vi "Setup.vi"(8 "error in (no error)":errorcluster, 11 "Scan Driver in":refnum<class "Scan Driver.lvclass">) -> (0 "error out":errorcluster, 3 "Scan Driver out":refnum<class "Scan Driver.lvclass">)   [LabVIEW 2017, in "Scan Driver.lvclass"]
doc: "GUI constructor for new Scan Driver instances. Call the component objects' Setup UI methods and use their GUIs to construct them too."
uses:
  Scan Driver.lvclass
  Scan Driver.lvclass/Scan Driver.ctl
  Scanners/Double Scanner/Double Scanner.lvclass
  C:/LabVIEW-programs/Scanners/Scanner/Scanner.lvclass
  Data Processing/Multi/Multi.lvclass
  C:/LabVIEW-programs/Data Processing/Aux Data Source/Aux Data Source.lvclass
  Readers/Reader/Reader.lvclass
  Scanners/Scanner/Scanner.lvclass
  File IO/File IO.lvclass
panel:
  in  "?":bool
  in  "Constant":dbl=1.0
  in  "Time between scans":dbl[unit]
  in  "Cancel":bool
  in  "# Scans":u32=1
  in  "Start Scan":bool
  in  "Aux Data Sources":T1
  # "Generic Scan Setup"
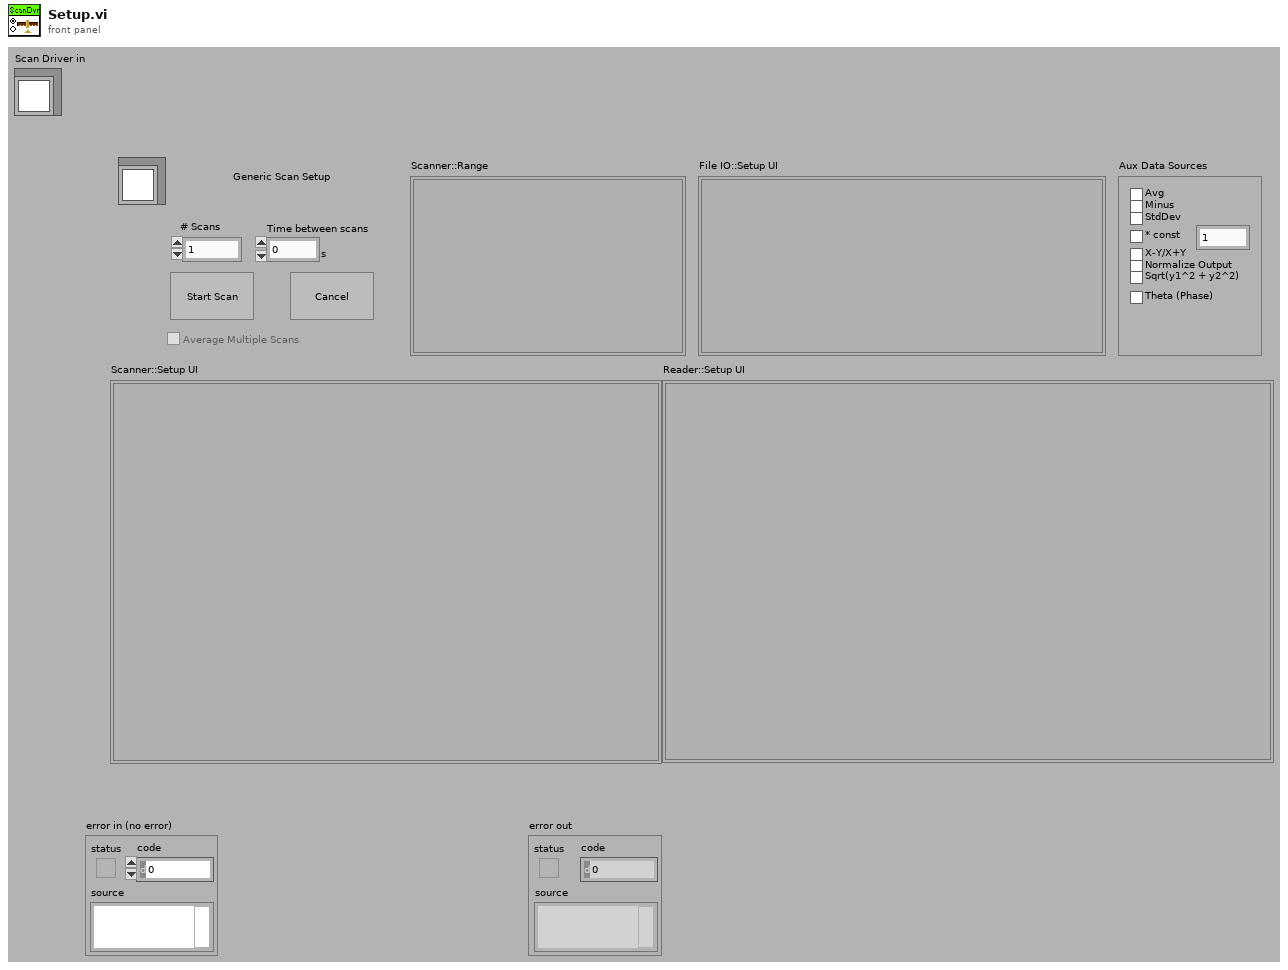
[diagram p1: front panel]
types:
  T1 = cluster{"Avg":bool, "Minus":bool, "StdDev":bool, "* const":bool, "X-Y/X+Y":bool, "Normalize Output":bool, "Sqrt(y1^2 + y2^2)":bool, "Theta (Phase)":bool}
  T2 = typedef "Scan Driver.lvclass/Scan Setup Mode.ctl" = enum32{"New Scan", "Load Last Scan", "Load Scan:"}
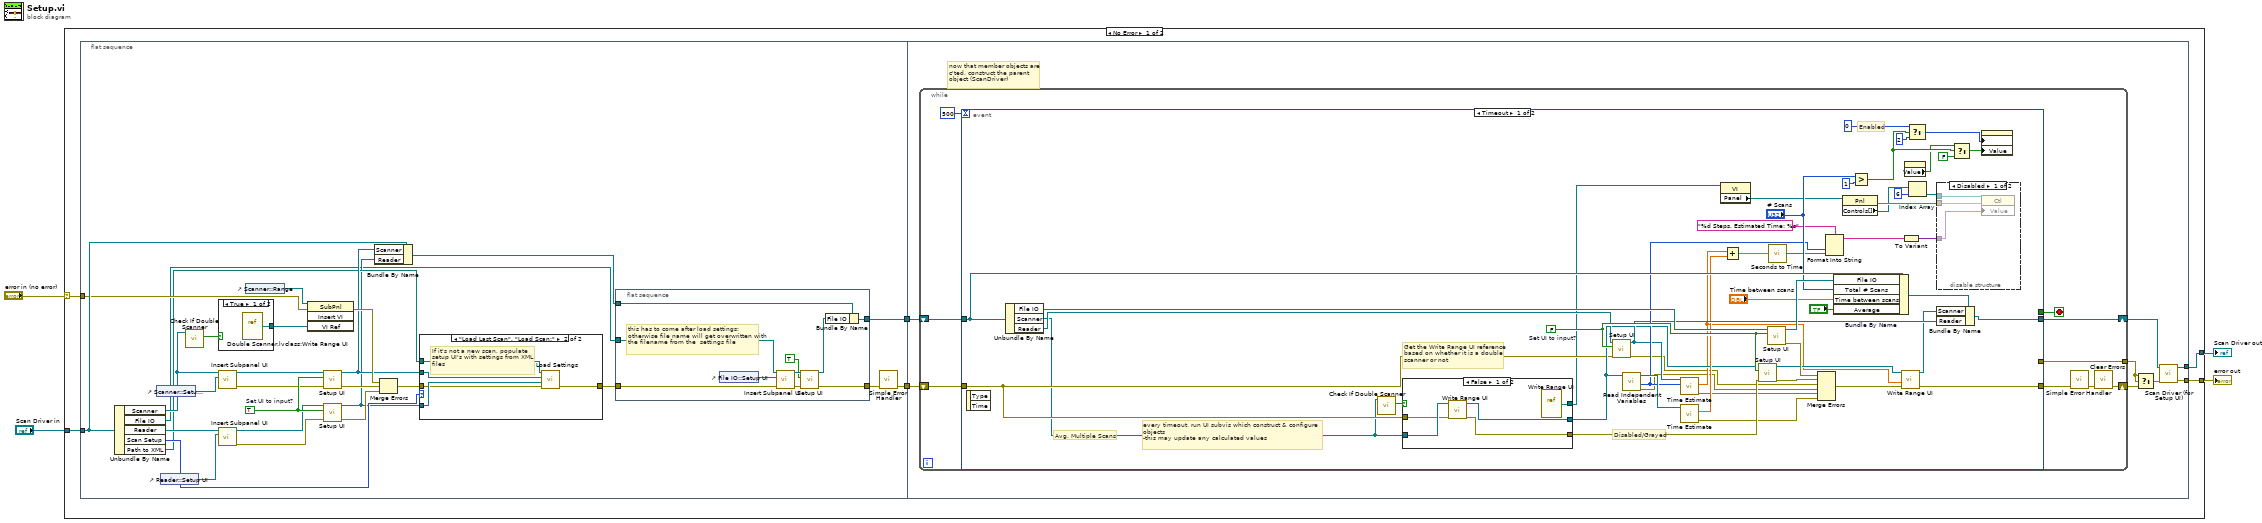
[diagram p0: block diagram]
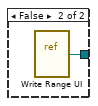
[diagram p3: hidden frame]
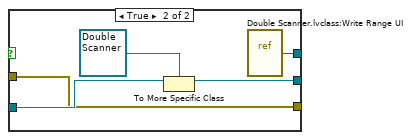
[diagram p5: hidden frame]
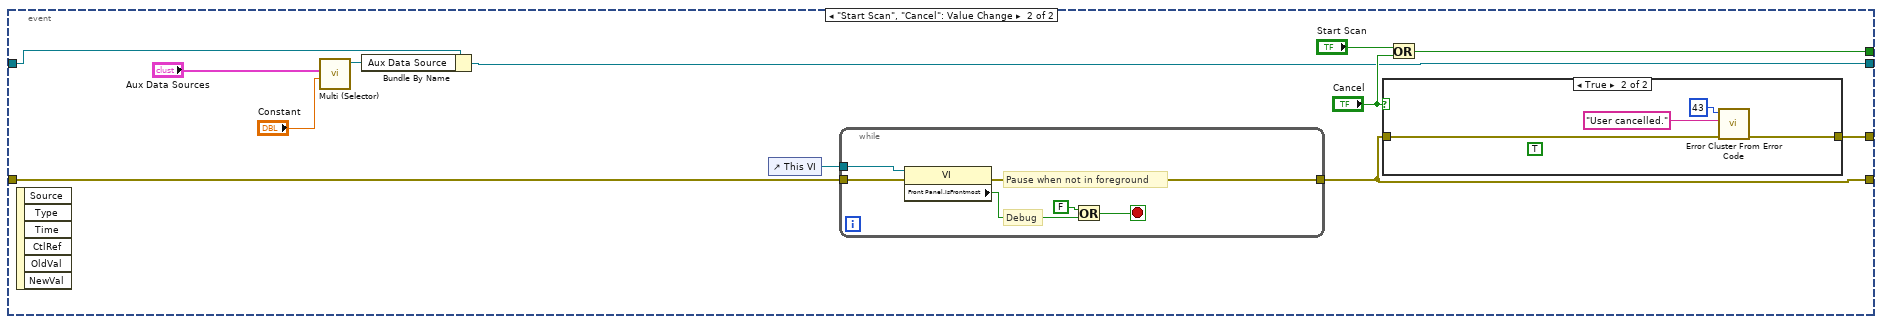
[diagram p6: hidden frame]
diagram:
  n1 = case shown="No Error" "error in (no error)" {
    selector: "error in (no error)" -> [w10 w160]
    tunnel: [w9 w160] -> w3
    tunnel: [w5 w159] -> w1
    tunnel: "Scan Driver in" -> [w8 w159]
    frame No Error {
      n2 = flat-sequence {
        tunnel: w10 -> [w27]
        tunnel: w8 -> [w30]
        tunnel: [w36] -> w7
        tunnel: [w14] -> w6
        tunnel: [w59] -> w9
        tunnel: w7 -> [w64]
        tunnel: w6 -> [w63]
        tunnel: [w57] -> w5
        frame #0 {
          w35 = TRUE  # Set UI to input?
          n3 = Unbundle By Name(w30) -> ("Scanner"=w22:refnum<class "Scanner.lvclass">, "File IO"=w13:refnum<class "File IO.lvclass">, "Reader"=w21:refnum<class "Reader.lvclass">, "Scan Setup"=w20:T2, "Path to XML"=w18:path)
          n4 = control-ref of="Scanner::Setup UI"() -> (w38:refnum<vi>)
          n5 = control-ref of="Reader::Setup UI"() -> (w37:refnum<vi>)
          n6 = call "Check If Double Scanner.vi"("Scanner in"=w22) -> ("Is Double Scanner?"=w29:bool)  [unwired: 10 in]
          n7 = case shown="True" w29 {
            tunnel: [w55 w56] -> w26
            frame True {
              n8 = vi-ref "Double Scanner.lvclass:Write Range UI.vi"() -> (w55:refnum<vi>)
            }
            frame False {
              n9 = vi-ref "Write Range UI.vi"() -> (w56:refnum<vi>)
            }
          }
          n10 = call "Insert Subpanel UI.vi"("Subpanel in"=w38, "LabVIEW Object"=w22) -> ("error out"=w32:errorcluster, "LabVIEW Object out"=w31:refnum<class "Scanner.lvclass">)  [unwired: 1 in, 7 out]
          n11 = call "Insert Subpanel UI.vi"("Subpanel in"=w37, "LabVIEW Object"=w21) -> ("error out"=w33:errorcluster, "LabVIEW Object out"=w34:refnum<class "Reader.lvclass">)  [unwired: 1 in, 7 out]
          n12 = control-ref of="Scanner::Range"() -> (w28:refnum<vi>)
          n13 = invoke on="Invoke Node" class="SubPnl" method="Insert VI"(reference=w28, error in=w27, "VI Ref"=w26) -> (error out=w25:errorcluster)  [unwired: 1 in, 3 out]
          n14 = call-dynamic "Setup UI.vi"("error in (no error)"=w32, "Set UI to input? (F)"=w35, "Scanner in"=w31) -> ("error out"=w24:errorcluster, "Scanner out"=w19:refnum<class "Scanner.lvclass">)  [unwired: 7 out]
          n15 = call-dynamic "Setup UI.vi"("error in (no error)"=w33, "Set UI to input? (F)"=w35, "Reader in"=w34) -> ("error out"=w23:errorcluster, "Reader out"=w17:refnum<class "Reader.lvclass">)  [unwired: 1 in, 6 out]
          n16 = Bundle By Name(cluster=w30, "Scanner"=w19, "Reader"=w17) -> (w15:refnum<class "Scan Driver.lvclass">)
          n17 = Merge Errors(w25, w24, w23) -> (w16:errorcluster)
          n18 = case shown="\"Load Last Scan\", \"Load Scan:\"" w20 {
            tunnel: w19 -> [_ w54]
            tunnel: w18 -> [_ w53]
            tunnel: w17 -> [_ w52]
            tunnel: w16 -> [w49 w51]
            tunnel: [w49 w50] -> w12
            frame "New Scan", Default {
            }
            frame "Load Last Scan", "Load Scan:" {
              # "If it's not a new scan, populate setup UI's with settings from XML files"
              n19 = call "Load Settings.vi"("error in (no error)"=w51, "Reader Object"=w52, "Scanner Object"=w54, "XML File Path"=w53) -> ("error out"=w50:errorcluster)  [unwired: 7 in]
            }
          }
          n20 = flat-sequence {
            tunnel: w15 -> [w46]
            tunnel: [w45] -> w14
            tunnel: w13 -> [w44]
            tunnel: w12 -> [w40]
            tunnel: [w39] -> w11
            frame #0 {
              # "this has to come after load settings; otherwise file name will get overwritten with the filename from the  settings file"
              n21 = control-ref of="File IO::Setup UI"() -> (w48:refnum<vi>)
              n22 = call "Insert Subpanel UI.vi"("error in (no error)"=w40, "Subpanel in"=w48, "LabVIEW Object"=w44) -> ("error out"=w43:errorcluster, "LabVIEW Object out"=w47:refnum<class "File IO.lvclass">)  [unwired: 7 out]
              n23 = call-dynamic "Setup UI.vi"("error in (no error)"=w43, "Set UI to input?"=TRUE, "File IO in"=w47) -> ("error out"=w39:errorcluster, "File IO out"=w42:refnum<class "File IO.lvclass">)  [unwired: 7 out]
              n24 = Bundle By Name(cluster=w46, "File IO"=w42) -> (w45:refnum<class "Scan Driver.lvclass">)
            }
          }
          n25 = call <vilib>:"Simple Error Handler.vi"("error in (no error)"=w11) -> ("error out"=w36:errorcluster)  [unwired: 1 in, 7 out]
        }
        frame #1 {
          # "now that member objects are\nc'ted, construct the parent\nobject (ScanDriver)"
          n26 = while {
            shift-right: [w72] -> w61
            shift-left: w64 -> [w73]
            shift-right: [w65] -> w58
            shift-left: w63 -> [w71]
            tunnel: [w67] -> w62
            stop <- w66 stop-if-true
            n27 = event shown="[0] Timeout" {
              selector: _ -> [_ _]
              dyn-events: _ -> [_ _]
              timeout: 500 -> [_ _]
              tunnel: w73 -> [w87 w138]
              tunnel: [w80 w136] -> w70
              tunnel: w71 -> [w121 w143]
              tunnel: [w122 w142] -> w65
              tunnel: [_ w144] -> w66
              tunnel: [_ w147] -> w67
              event Timeout {
                w119 = FALSE  # Set UI to input?
                # "Get the Write Range UI reference\nbased on whether it is a double\nscanner or not"
                # "Avg. Multiple Scans"
                # "Disabled/Grayed"
                # "Enabled"
                # "every timeout, run UI subvis which construct & configure objects\n-this may update any calculated values"
                n28 = event-data() -> ()  [unwired: 3 out]
                n29 = Unbundle By Name(w121) -> ("File IO"=w118:refnum<class "File IO.lvclass">, "Scanner"=w85:refnum<class "Scanner.lvclass">, "Reader"=w113:refnum<class "Reader.lvclass">)
                n30 = call "Check If Double Scanner.vi"("Scanner in"=w85) -> ("Is Double Scanner?"=w86:bool)  [unwired: 10 in]
                n31 = case shown="False" w86 {
                  tunnel: w85 -> [w130 w135]
                  tunnel: [w129 w132] -> w89
                  tunnel: [w128 w131] -> w88
                  tunnel: w87 -> [w127 w131]
                  tunnel: [w126 w133] -> w84
                  frame False {
                    n32 = call-dynamic "Write Range UI.vi"("error in (no error)"=w127, "Scanner in"=w130) -> ("error out"=w128:errorcluster, "Scanner out"=w129:refnum<class "Scanner.lvclass">)  [unwired: 2 in, 6 out]
                    n33 = vi-ref "Write Range UI.vi"() -> (w126:refnum<vi>)
                  }
                  frame True {
                    n34 = To More Specific Class(target class=refnum<class "Double Scanner.lvclass"> refnum ("Double Scanner.lvclass"), reference=w135) -> (specific class reference=w132:refnum<class "Double Scanner.lvclass">)  [unwired: 1 in, 1 out]
                    n35 = vi-ref "Double Scanner.lvclass:Write Range UI.vi"() -> (w133:refnum<vi>)
                  }
                }
                n36 = call-dynamic "Setup UI.vi"("error in (no error)"=w87, "Set UI to input? (F)"=w119, "Reader in"=w113) -> ("error out"=w77:errorcluster, "Reader out"=w93:refnum<class "Reader.lvclass">)  [unwired: 1 in, 6 out]
                n37 = call-dynamic "Read Independent Variables.vi"("Scanner.lvclass in"=w89) -> ("error out"=w76:errorcluster, "size"=w94:i32, "Scanner.lvclass out"=w95:refnum<class "Scanner.lvclass">)  [unwired: 1 in, 7 out]
                n38 = call-dynamic "Time Estimate.vi"("Points"=w94, "Reader in"=w93) -> ("error out"=w75:errorcluster, "time"=w78:dbl[unit])  [unwired: 7 in, 1 out]
                n39 = call-dynamic "Time Estimate.vi"("Scanner.lvclass"=w95) -> ("error out"=w74:errorcluster, "time"=w92:dbl[unit])  [unwired: 7 in, 2 out]
                n40 = property class="VI"(reference=w84) -> ("Panel"=w99:refnum<vi>)  [unwired: 1 in, 2 out]
                n41 = Add(x=w78, y=w92) -> (x+y=w91:dbl[unit])
                n42 = call-dynamic "Setup UI.vi"("error in (no error)"=w88, "Set UI to input? (F)"=w119, "Scanner in"=w89) -> ("error out"=w114:errorcluster, "Scanner out"=w83:refnum<class "Scanner.lvclass">)  [unwired: 7 out]
                n43 = call-dynamic "Setup UI.vi"("Set UI to input?"=w119, "File IO in"=w118) -> ("error out"=w116:errorcluster, "File IO out"=w117:refnum<class "File IO.lvclass">)  [unwired: 1 in, 7 out]
                n44 = call "Seconds to Time.vi"("Seconds"=w91) -> ("Time"=w96:string)
                n45 = Merge Errors(w116, w114, w77, w76, w75, w74) -> (w81:errorcluster)
                n46 = Format Into String(format string="%d Steps, Estimated Time: %s", w94, w96) -> (resulting string=w90:string)  [unwired: 2 in, 1 out]
                n47 = Bundle By Name(cluster=w121, "File IO"=w117, "Total # Scans"="# Scans", "Time between scans"="Time between scans", "Average"="?") -> (w120:refnum<class "Scan Driver.lvclass">)
                n48 = property class="Pnl"(reference=w99) -> (error out=w100:errorcluster, "Controls[]"=w98:refnum<vi>[])  [unwired: 1 in, 1 out]
                n49 = Greater?(x="# Scans", y=1) -> (0:w107:bool)
                n50 = call-dynamic "Write Range UI.vi"("error in (no error)"=w81, "Reader Time"=w78, "Scanner in"=w83) -> ("error out"=w80:errorcluster, "Scanner out"=w82:refnum<class "Scanner.lvclass">)  [unwired: 7 in]
                n51 = To Variant(anything=w90) -> (Variant=w79:variant)
                n52 = property class="Bool (strict)"() -> ("Value"=w104:bool)  [unwired: 2 in, 2 out]
                n53 = Select(t=0, s=w107, f=2) -> (s? t:f=w110:i32)
                n54 = Index Array(array=w98, index=6) -> (element=w101:refnum<vi>)
                n55 = disable-structure shown="Disabled" {
                  disable-tunnel: w101 -> [w125 _]
                  disable-tunnel: w100 -> [w124 _]
                  disable-tunnel: w79 -> [w123 _]
                  frame Disabled {
                    n56 = property class="Ctl"(reference=w125, error in=w124, "Value"=w123) -> ()  [unwired: 2 out]
                  }
                  frame Enabled {
                  }
                }
                n57 = Bundle By Name(cluster=w120, "Scanner"=w82, "Reader"=w93) -> (w122:refnum<class "Scan Driver.lvclass">)
                n58 = Select(t=w104, s=w107, f=FALSE) -> (s? t:f=w105:bool)
                n59 = property class="Bool (strict)"("DisabledEnum"=w110, "Value"=w105) -> ()  [unwired: 2 in, 2 out]
              }
              event "Start Scan", "Cancel": Value Change {
                n60 = event-data() -> ()  [unwired: 7 out]
                n61 = call "Multi (Selector).vi"("Constant"="Constant", "Aux Data Sources"="Aux Data Sources") -> ("Multi out"=w141:refnum<class "Multi.lvclass">)  [unwired: 8 in, 1 out]
                n62 = Bundle By Name(cluster=w143, "Aux Data Source"=w141) -> (w142:refnum<class "Scan Driver.lvclass">)
                n63 = control-ref of="This VI"() -> (w137:refnum<vi>)
                n64 = while {
                  tunnel: [w153] -> w136
                  tunnel: w138 -> [w149]
                  tunnel: w137 -> [w148]
                  stop <- w152 stop-if-true
                  # "Pause when not in foreground"
                  # "Debug"
                  n65 = property class="VI"(reference=w148, error in=w149) -> (error out=w153:errorcluster, "Front Panel.IsFrontmost"=w150:bool)  [unwired: 1 out]
                  n66 = Or(x=FALSE, y=w150) -> (x .or. y?=w152:bool)
                }
                n67 = case shown="True" "Cancel" {
                  tunnel: [w154 w158] -> w147
                  tunnel: w136 -> [w154 w155]
                  frame False {
                  }
                  frame True {
                    (unwired) TRUE ("status")
                    n68 = call <vilib>:"Error Cluster From Error Code.vi"("error in (no error)"=w155, "error message (\"\")"="User cancelled." ("source"), "error code (0)"=43 ("code")) -> ("error out"=w158:errorcluster)  [unwired: 2 in, 4 out]
                  }
                }
                n69 = Or(x="Start Scan", y="Cancel") -> (x .or. y?=w144:bool)
              }
            }
            n70 = call <vilib>:"Simple Error Handler.vi"("error in (no error)"=w70) -> ("error out"=w69:errorcluster)  [unwired: 1 in, 7 out]
            n71 = call <vilib>:"Clear Errors.vi"("error in (no error)"=w69) -> ("error out"=w72:errorcluster)  [unwired: 1 in, 5 out]
          }
          n72 = Select(t=w62, s=w62, f=w61) -> (s? t:f=w60:errorcluster)
          n73 = call "Scan Driver (for Setup UI).vi"("error in (no error)"=w60, "Scan Driver.lvclass in"=w58) -> ("error out"=w59:errorcluster, "Scan Driver.lvclass out"=w57:refnum<class "Scan Driver.lvclass">)  [unwired: 1 in, 7 out]
        }
      }
    }
    frame Error {
    }
  }
  "error out" <- w3
  "Scan Driver out" <- w1
